vi "Stop Core.vi"(10 "最终错误代码":i32, 11 "操作者框架输入":refnum<class "操作者框架.lvclass">) -> (3 "操作者框架输出":refnum<class "操作者框架.lvclass">)   [LabVIEW 2013, in "操作者框架.lvlib" / "操作者框架.lvclass"]
uses:
  <vilib>/ActorFramework/Actor/Actor.lvclass
  <vilib>/ActorFramework/Stop Msg/Stop Msg.lvclass/Stop Msg.ctl
  <vilib>/ActorFramework/Message Enqueuer/Message Enqueuer.lvclass/Message Enqueuer.ctl
  <vilib>/ActorFramework/Stop Msg/Send Emergency Stop.vi
  <vilib>/ActorFramework/Stop Msg/Send Normal Stop.vi
  <vilib>/ActorFramework/Message Enqueuer/Enqueue Critical.vi
  <vilib>/ActorFramework/Message Enqueuer/Enqueue.vi
  <vilib>/ActorFramework/Message Priority Queue/Priority Enqueue.vi
  <vilib>/ActorFramework/Stop Msg/Stop Msg.lvclass
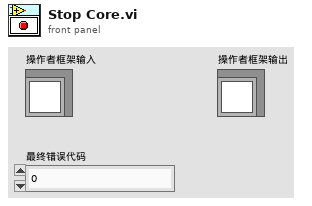
[diagram p1: front panel]
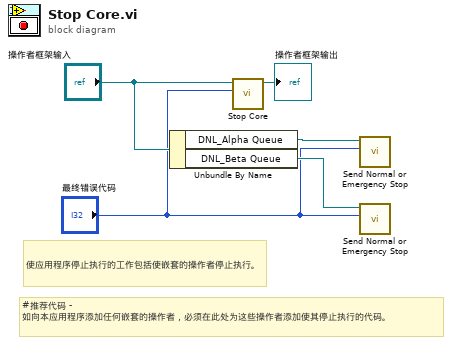
[diagram p0: block diagram]
diagram:
  # "#推荐代码 - 如向本应用程序添加任何嵌套的操作者，必须在此处为这些操作者添加使其停止执行的代码。"
  # "使应用程序停止执行的工作包括使嵌套的操作者停止执行。"
  n1 = Unbundle By Name("操作者框架输入") -> ("DNL_Alpha Queue"=w3:refnum<class "Message Enqueuer.lvclass">, "DNL_Beta Queue"=w2:refnum<class "Message Enqueuer.lvclass">)
  n2 = call-parent "Stop Core.vi"("final error code"="最终错误代码", "Actor in"="操作者框架输入") -> ("Actor out"=→"操作者框架输出":refnum<class "操作者框架.lvclass">)  [unwired: 9 in]
  n3 = call <vilib>:"Send Normal or Emergency Stop.vi"("final error code"="最终错误代码", "Message Enqueuer"=w3) -> ()  [unwired: 9 in, 1 out]
  n4 = call <vilib>:"Send Normal or Emergency Stop.vi"("final error code"="最终错误代码", "Message Enqueuer"=w2) -> ()  [unwired: 9 in, 1 out]
